vi "FGV Interference.vi"(0 "TestKonfig":T5={"TestKonfig H2O"={"Modus"=0, "Komponente:"=0, "Eingangs Konzentration:"=120.0, "Einheit"=enum."ppm", "Anzahl Stufen"=0.0, "Zeitdauer Stufen"=0.0, "Max Fehler"=0.0, "zusätzliche Zeitdauer Erster Punkt"=30.0, "Punkte umkehren"=FALSE, "Stufen Tabelle"=[], "HovaCAL Flow Input Cluster"={"HovaCAL Flow Input Cluster"=0.0}, "HovaCAL Temperature"=[]}, "TestKonfig Interferent"={"MFC1"=enum."MFC 1", "Eingangs Konzentration MFC1"=120.0, "Einheit MFC1 Eingang"=enum."ppm", "Ausgangs Konzentration MFC1"=120.0, "Einheit MFC1 Ausgang"=enum."ppm", "MFC2"=0, "Referenz-Interferent:"=0, "Gasflaschen Nr MFC2"="", "Eingangs Konzentration MFC2"=120.0, "Einheit MFC2 Eingang"=enum."ppm", "Accuracy MFC2"="", "Ausgangs Konzentration MFC2"=120.0, "Einheit MFC2 Ausgang"=enum."ppm", "MFC3"=1, "Kontroll-Interferent:"=0, "Gasflaschen Nr MFC3"="", "Accuracy MFC3"="", "Eingangs Konzentration MFC3"=120.0, "Einheit MFC3 Eingang"=enum."ppm", "Ausgangs Konzentration MFC3"=120.0, "Einheit MFC3 Ausgang"=enum."ppm", "Gasflasche MFC2"=0, "Gasflasche MFC3"=0}} {"TestKonfig Interferent"."Gasflasche MFC3" items=["----"=10000, "IAG NH3 3000"=0, "IAG NH3 200"=1, "IAG NH3 2000"=2, "IAG MG"=3, "IAG O2"=4]; "TestKonfig Interferent"."Gasflasche MFC2" items=["----"=10000, "IAG NH3 3000"=0, "IAG NH3 200"=1, "IAG NH3 2000"=2, "IAG MG"=3, "IAG O2"=4]; "TestKonfig Interferent"."Eingangs Konzentration MFC1" min=0.0; "TestKonfig Interferent"."Ausgangs Konzentration MFC1" min=0.0; "TestKonfig Interferent"."MFC2" items=["MFC 2", "MFC 3", "MFC 4", "MFC 5"]; "TestKonfig Interferent"."MFC3" items=["MFC 2", "MFC 3", "MFC 4", "MFC 5"]; "TestKonfig Interferent"."Ausgangs Konzentration MFC3" min=0.0; "TestKonfig Interferent"."Eingangs Konzentration MFC3" min=0.0; "TestKonfig Interferent"."Ausgangs Konzentration MFC2" min=0.0; "TestKonfig Interferent"."Eingangs Konzentration MFC2" min=0.0; "TestKonfig H2O"."HovaCAL Temperature" format="%.2f"; "TestKonfig H2O"."HovaCAL Flow Input Cluster"."HovaCAL Flow Input Cluster" format="%.2f"; "TestKonfig H2O"."Eingangs Konzentration:" min=0.0; "TestKonfig H2O"."zusätzliche Zeitdauer Erster Punkt" min=30 step=1 format="%#_5g"; "TestKonfig H2O"."Zeitdauer Stufen" format="%#_5g"; "TestKonfig H2O"."Max Fehler" format="%#_5g"; "TestKonfig H2O"."Anzahl Stufen" format="%#_5g"; "TestKonfig H2O"."Modus" items=["Messen", "CG zu Entnahmestelle"]}, 1 "TestSetting":T1={"Bearbeiter:"="", "Pfad:"=path "D:/IAG_Data/Log", "Textname:"="", "Analysator"=""}, 2 "Ergebnis":T4 caption="Ergebnis Cluster", 5 "Ergebnis":sgl[](array[numeric]), 7 "Einheiten":string[](array[string]), 9 "Tabelle":T3[][](array[typedef]), 11 "error in (no error)":errorcluster caption="Fehler (Eingang, kein Fehler)", 12 "Aktion FGV Interference":T15) -> (3 "TestSetting":T1={"Bearbeiter:"="", "Pfad:"=path "D:/IAG_Data/Log", "Textname:"="", "Analysator"=""}, 4 "TestKonfig":T5={"TestKonfig H2O"={"Modus"=0, "Komponente:"=0, "Eingangs Konzentration:"=120.0, "Einheit"=enum."ppm", "Anzahl Stufen"=0.0, "Zeitdauer Stufen"=0.0, "Max Fehler"=0.0, "zusätzliche Zeitdauer Erster Punkt"=30.0, "Punkte umkehren"=FALSE, "Stufen Tabelle"=[], "HovaCAL Flow Input Cluster"={"HovaCAL Flow Input Cluster"=0.0}, "HovaCAL Temperature"=[]}, "TestKonfig Interferent"={"MFC1"=enum."MFC 1", "Eingangs Konzentration MFC1"=120.0, "Einheit MFC1 Eingang"=enum."ppm", "Ausgangs Konzentration MFC1"=120.0, "Einheit MFC1 Ausgang"=enum."ppm", "MFC2"=0, "Referenz-Interferent:"=0, "Gasflaschen Nr MFC2"="", "Eingangs Konzentration MFC2"=120.0, "Einheit MFC2 Eingang"=enum."ppm", "Accuracy MFC2"="", "Ausgangs Konzentration MFC2"=120.0, "Einheit MFC2 Ausgang"=enum."ppm", "MFC3"=1, "Kontroll-Interferent:"=0, "Gasflaschen Nr MFC3"="", "Accuracy MFC3"="", "Eingangs Konzentration MFC3"=120.0, "Einheit MFC3 Eingang"=enum."ppm", "Ausgangs Konzentration MFC3"=120.0, "Einheit MFC3 Ausgang"=enum."ppm", "Gasflasche MFC2"=0, "Gasflasche MFC3"=0}} {"TestKonfig Interferent"."Gasflasche MFC3" items=["----"=10000, "IAG NH3 3000"=0, "IAG NH3 200"=1, "IAG NH3 2000"=2, "IAG MG"=3, "IAG O2"=4]; "TestKonfig Interferent"."Gasflasche MFC2" items=["----"=10000, "IAG NH3 3000"=0, "IAG NH3 200"=1, "IAG NH3 2000"=2, "IAG MG"=3, "IAG O2"=4]; "TestKonfig Interferent"."Eingangs Konzentration MFC1" min=0.0; "TestKonfig Interferent"."Ausgangs Konzentration MFC1" min=0.0; "TestKonfig Interferent"."MFC2" items=["MFC 2", "MFC 3", "MFC 4", "MFC 5"]; "TestKonfig Interferent"."MFC3" items=["MFC 2", "MFC 3", "MFC 4", "MFC 5"]; "TestKonfig Interferent"."Ausgangs Konzentration MFC3" min=0.0; "TestKonfig Interferent"."Eingangs Konzentration MFC3" min=0.0; "TestKonfig Interferent"."Ausgangs Konzentration MFC2" min=0.0; "TestKonfig Interferent"."Eingangs Konzentration MFC2" min=0.0; "TestKonfig H2O"."HovaCAL Temperature" format="%.2f"; "TestKonfig H2O"."HovaCAL Flow Input Cluster"."HovaCAL Flow Input Cluster" format="%.2f"; "TestKonfig H2O"."Eingangs Konzentration:" min=0.0; "TestKonfig H2O"."zusätzliche Zeitdauer Erster Punkt" min=30 step=1 format="%#_5g"; "TestKonfig H2O"."Zeitdauer Stufen" format="%#_5g"; "TestKonfig H2O"."Max Fehler" format="%#_5g"; "TestKonfig H2O"."Anzahl Stufen" format="%#_5g"; "TestKonfig H2O"."Modus" items=["Messen", "CG zu Entnahmestelle"]}, 6 "Ergebnis":T4, 8 "Einheiten":string[](array[string]), 10 "Tabelle":T3[][](array[typedef]), 15 "error out":errorcluster caption="Fehler (Ausgang)")   [LabVIEW 2020, in "EPA 1065.lvlib" / "HovaCAL Interference verificaton.lvlib"]
uses:
  HovaCAL Interference verificaton.lvlib
  Aktion FGV Interference.ctl
  TestKonfig.ctl
  TestKonfig H2O.ctl
  Modus.ctl
  Linearisierung V2/SpanEinstellungen/Einheit.ctl
  Linearisierung V2/Gasteiler/Stufen Tabelle.ctl
  Linearisierung V2/Gasteiler/HovaCAL_Interface/Controls/Flow Einstellung.ctl
  Linearisierung V2/Gasteiler/HovaCAL_Interface/Controls/Temp Sollwerte Anzeige.ctl
  TestKonfig Interferents.ctl
  MFCAuswahl.ctl
  Seiten/System Einstellungen V2/Gasflasche Auswahl.ctl
  Ergebnis.ctl
  Visualisierungs Elemente/String - Ausgabefeld.ctl
  TestSetting.ctl
  Seiten/System Einstellungen V2/Analysatoren.ctl
  Allgemein/allgemeine Sub-VIs.lvlib
  Seiten/System Einstellungen V2/System Einstellungen V2.lvlib
  Linearisierung V2/SpanEinstellungen/SpanEinstellungen.lvlib
  Linearisierung V2/Gasteiler/Gasteiler.lvlib
  Linearisierung V2/Gasteiler/HovaCAL_Interface/Controls/Controls.lvlib
panel:
  # "sec"
  # "%"
  # "sec"
  # "sec"
  # "%"
  # "sec"
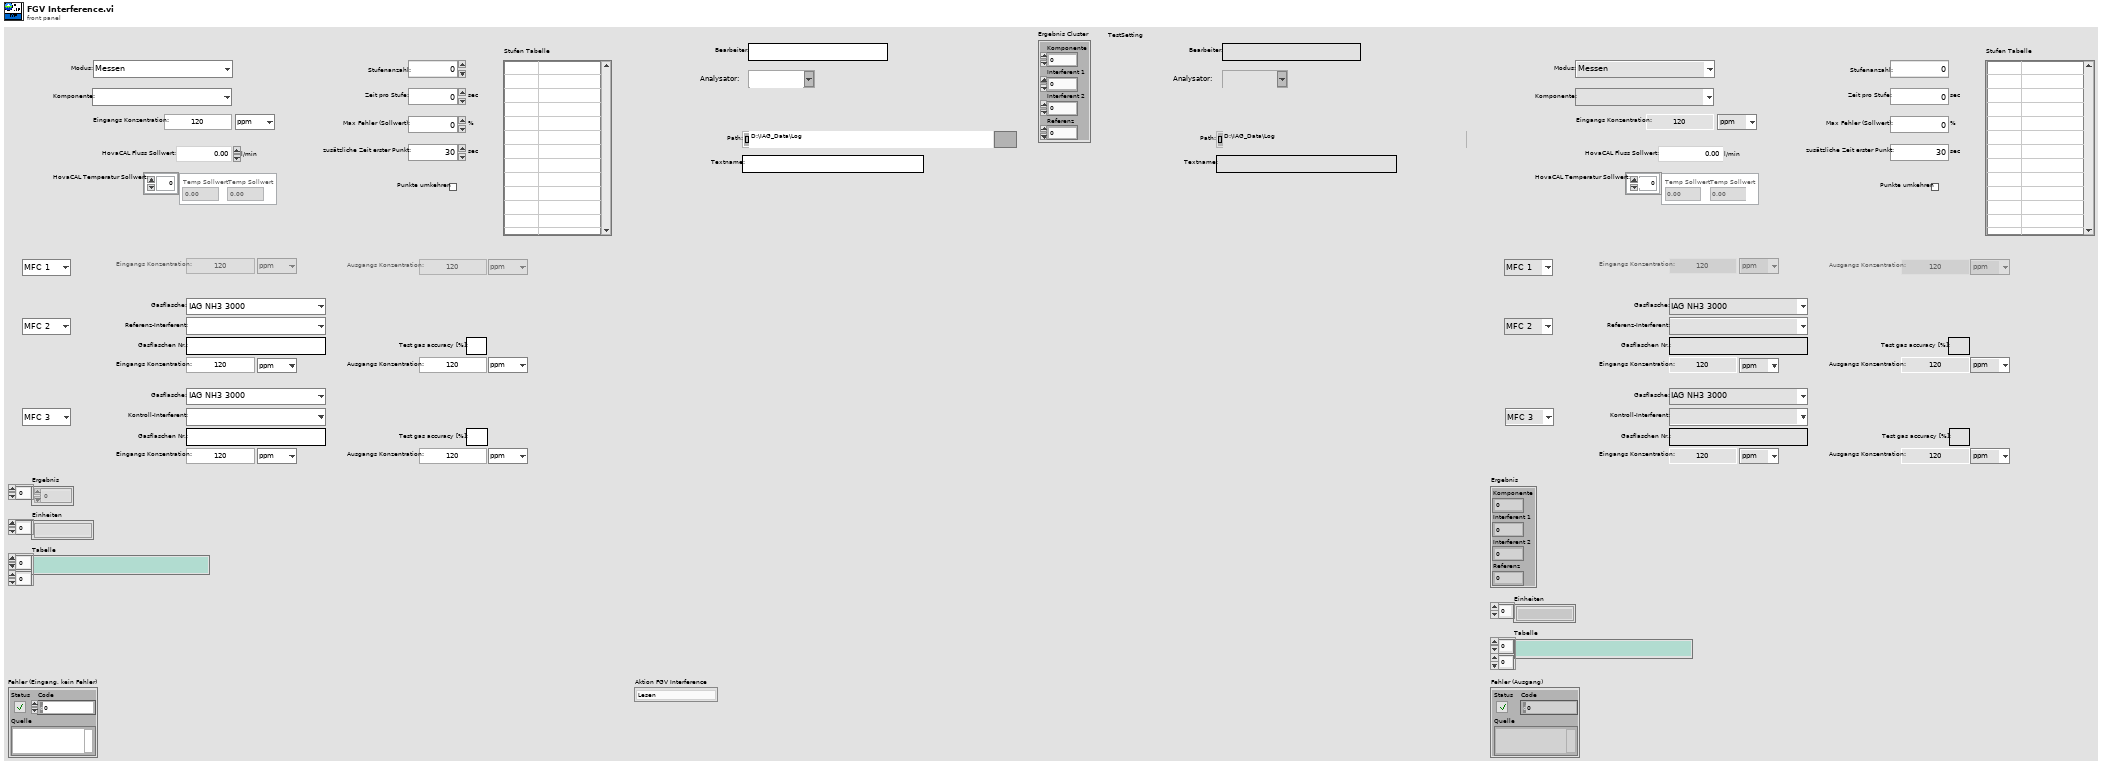
[diagram p1: front panel]
types:
  T1 = typedef "EPA 1065.lvlib/HovaCAL Interference verificaton.lvlib/TestSetting.ctl" = cluster{"Bearbeiter:":string, "Pfad:":path, "Textname:":string, "Analysator":T2}
  T2 = typedef "System Einstellungen V2.lvlib/Analysatoren.ctl" = string
  T3 = typedef "String - Ausgabefeld.ctl" = string
  T4 = typedef "EPA 1065.lvlib/HovaCAL Interference verificaton.lvlib/Ergebnis.ctl" = cluster{"Komponente":sgl, "Interferent 1":sgl, "Interferent 2":sgl, "Referenz":sgl}
  T5 = typedef "EPA 1065.lvlib/HovaCAL Interference verificaton.lvlib/TestKonfig.ctl" = cluster{"TestKonfig H2O":T6, "TestKonfig Interferent":T12}
  T6 = typedef "EPA 1065.lvlib/HovaCAL Interference verificaton.lvlib/TestKonfig H2O.ctl" = cluster{"Modus":T7, "Komponente:":u16, "Eingangs Konzentration:":dbl, "Einheit":T8, "Anzahl Stufen":sgl, "Zeitdauer Stufen":sgl, "Max Fehler":sgl, "zusätzliche Zeitdauer Erster Punkt":sgl, "Punkte umkehren":bool, "Stufen Tabelle":T9, "HovaCAL Flow Input Cluster":T10, "HovaCAL Temperature":T11}
  T7 = typedef "EPA 1065.lvlib/HovaCAL Interference verificaton.lvlib/Modus.ctl" = u16
  T8 = typedef "Linearisierung v2.lvlib/SpanEinstellungen.lvlib/Einheit.ctl" = enum16{"ppm", "%"}
  T9 = typedef "Linearisierung v2.lvlib/Gasteiler.lvlib/Stufen Tabelle.ctl" = string[][]
  T10 = typedef "Linearisierung v2.lvlib/Gasteiler.lvlib/HovaCAL_Interface.lvlib/Controls.lvlib/Flow Einstellung.ctl" = cluster{"HovaCAL Flow Input Cluster":dbl}
  T11 = typedef "Linearisierung v2.lvlib/Gasteiler.lvlib/HovaCAL_Interface.lvlib/Controls.lvlib/Temp Sollwerte Anzeige.ctl" = dbl[]
  T12 = typedef "EPA 1065.lvlib/HovaCAL Interference verificaton.lvlib/TestKonfig Interferents.ctl" = cluster{"MFC1":enum16{"MFC 1"}, "Eingangs Konzentration MFC1":dbl, "Einheit MFC1 Eingang":T8, "Ausgangs Konzentration MFC1":dbl, "Einheit MFC1 Ausgang":T8, "MFC2":T13, "Referenz-Interferent:":u16, "Gasflaschen Nr MFC2":string, "Eingangs Konzentration MFC2":dbl, "Einheit MFC2 Eingang":T8, "Accuracy MFC2":string, "Ausgangs Konzentration MFC2":dbl, "Einheit MFC2 Ausgang":T8, "MFC3":T13, "Kontroll-Interferent:":u16, "Gasflaschen Nr MFC3":string, "Accuracy MFC3":string, "Eingangs Konzentration MFC3":dbl, "Einheit MFC3 Eingang":T8, "Ausgangs Konzentration MFC3":dbl, "Einheit MFC3 Ausgang":T8, "Gasflasche MFC2":T14, "Gasflasche MFC3":T14}
  T13 = typedef "EPA 1065.lvlib/HovaCAL Interference verificaton.lvlib/MFCAuswahl.ctl" = u16
  T14 = typedef "System Einstellungen V2.lvlib/Gasflasche Auswahl.ctl" = u16
  T15 = typedef "EPA 1065.lvlib/HovaCAL Interference verificaton.lvlib/Aktion FGV Interference.ctl" = enum16{"Lesen", "TestKonfig", "TestSetting", "Einheiten", "Ergebnis", "Laden", "Tabelle", "Speichern", "löschen"}
  T16 = enum16{"open", "replace", "create", "open or create", "replace or create", "replace or create with confirmation"}
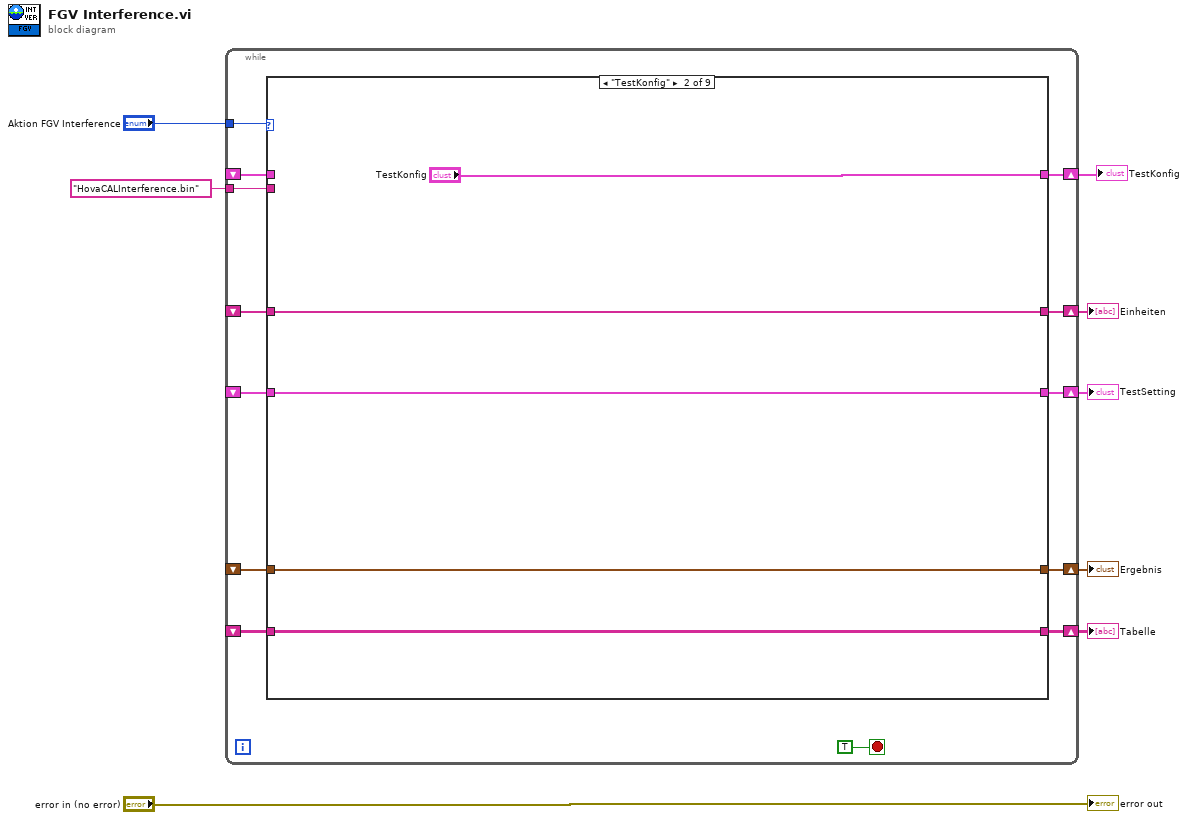
[diagram p0: block diagram]
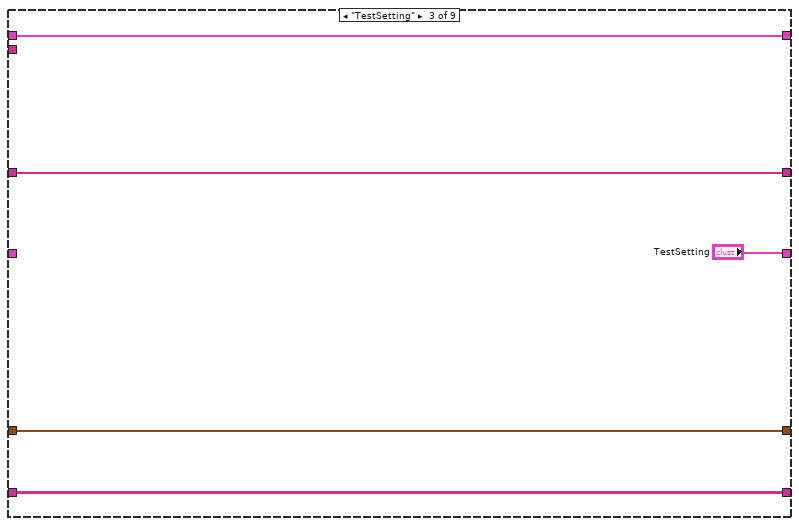
[diagram p3: hidden frame]
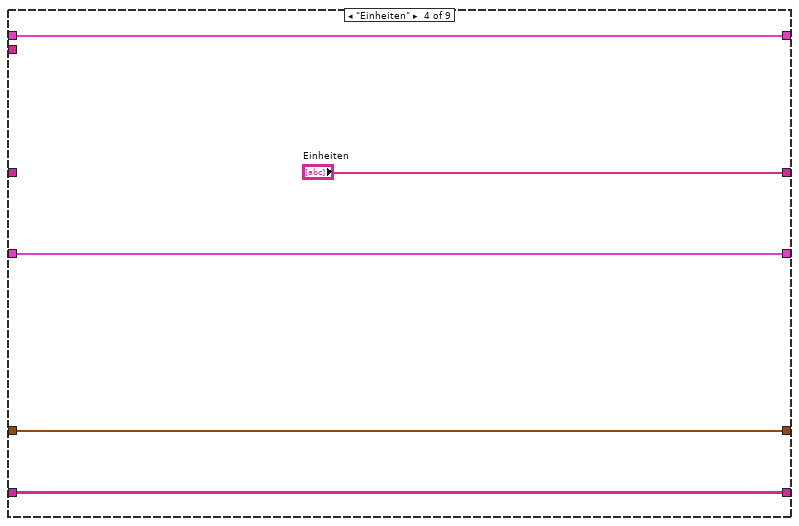
[diagram p4: hidden frame]
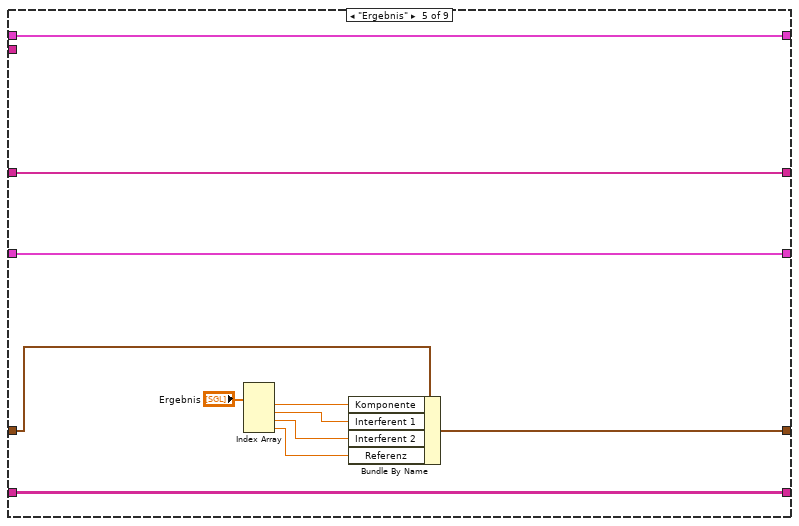
[diagram p5: hidden frame]
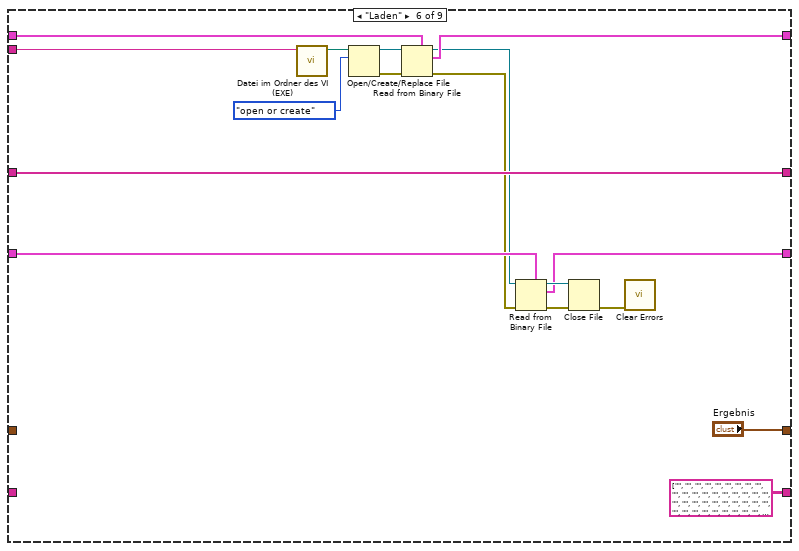
[diagram p6: hidden frame]
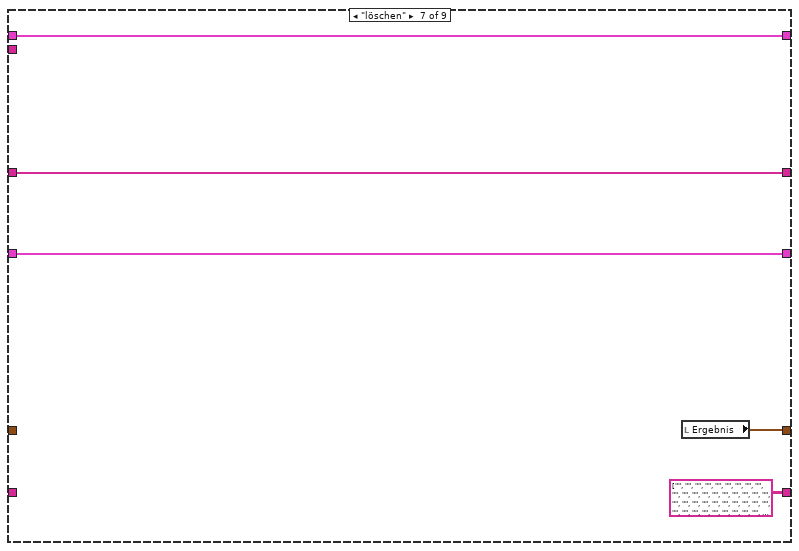
[diagram p7: hidden frame]
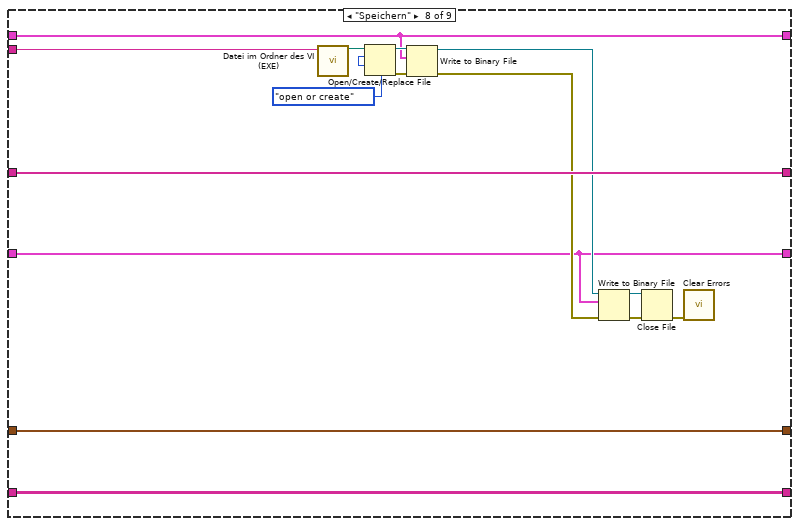
[diagram p8: hidden frame]
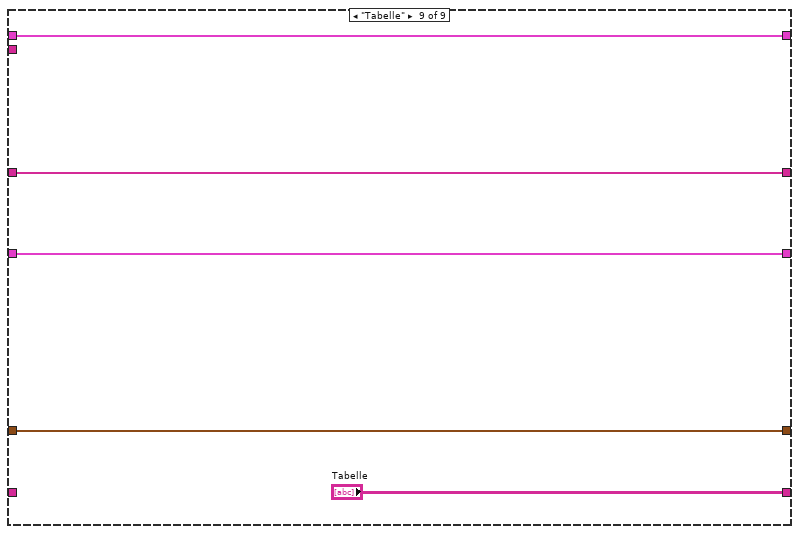
[diagram p9: hidden frame]
diagram:
  n1 = while {
    tunnel: "Aktion FGV Interference" -> [w20]
    shift-right: [w21] -> w6
    shift-left: _ -> [w19]
    shift-right: [w17] -> w5
    shift-left: _ -> [w16]
    shift-right: [w15] -> w4
    shift-left: _ -> [w14]
    shift-right: [w13] -> w3
    shift-left: _ -> [w12]
    shift-right: [w11] -> w2
    shift-left: _ -> [w10]
    tunnel: "HovaCALInterference.bin" ("Dateiname") -> [w9]
    stop <- TRUE stop-if-true
    n2 = case shown="\"TestKonfig\"" w20 {
      tunnel: [w26 "TestKonfig" w33 w41 w52 w61 w72 w82 w92] -> w21
      tunnel: w19 -> [w26 _ w33 w41 w52 w62 w72 w82 w92]
      tunnel: [w25 w30 w36 w40 w47 "Ergebnis" w71 w89 w94] -> w17
      tunnel: w16 -> [w25 w30 w36 w40 w50 _ _ w89 w94]
      tunnel: [w24 w29 w35 "Einheiten" w49 w68 w74 w88 w93] -> w15
      tunnel: w14 -> [w24 w29 w35 _ w49 w68 w74 w88 w93]
      tunnel: [w23 w28 w34 w38 w48 T3[][] [["", "", "", "", "", "", "", "", "", "", ""], ["", "", "", "", "", "", "", "", "", "", ""], ["", "", "", "", "", "", "", "", "", "", ""], ["", "", "", "", "", "", "", "", "", "", ""], ["", "", "", "", "", "", "", "", "", "", ""], ["", "", "", "", "", "", "", "", "", "", ""], ["", "", "", "", "", "", "", "", "", "", ""], ["", "", "", "", "", "", "", "", "", "", ""], ["", "", "", "", "", "", "", "", "", "", ""], ["", "", "", "", "", "", "", "", "", "", ""], ["", "", "", "", "", "", "", "", "", "", ""]] ("Tabelle") T3[][] [["", "", "", "", "", "", "", "", "", "", ""], ["", "", "", "", "", "", "", "", "", "", ""], ["", "", "", "", "", "", "", "", "", "", ""], ["", "", "", "", "", "", "", "", "", "", ""], ["", "", "", "", "", "", "", "", "", "", ""], ["", "", "", "", "", "", "", "", "", "", ""], ["", "", "", "", "", "", "", "", "", "", ""], ["", "", "", "", "", "", "", "", "", "", ""], ["", "", "", "", "", "", "", "", "", "", ""], ["", "", "", "", "", "", "", "", "", "", ""], ["", "", "", "", "", "", "", "", "", "", ""]] ("Tabelle") w87 "Tabelle"] -> w13
      tunnel: w12 -> [w23 w28 w34 w38 w48 _ _ w87 _]
      tunnel: [w22 w27 "TestSetting" w37 w46 w56 w70 w76 w91] -> w11
      tunnel: w10 -> [w22 w27 _ w37 w46 w57 w70 w76 w91]
      tunnel: w9 -> [_ _ _ _ _ w53 _ w75 _]
      frame "Lesen", Default {
      }
      frame "TestKonfig" {
      }
      frame "TestSetting" {
      }
      frame "Einheiten" {
      }
      frame "Ergebnis" {
        n3 = Index Array(array="Ergebnis") -> (element #1=w45:sgl, element #2=w44:sgl, element #3=w43:sgl, element #4=w42:sgl)  [unwired: 4 in]
        n4 = Bundle By Name(cluster=w50, "Komponente"=w45, "Interferent 1"=w44, "Interferent 2"=w43, "Referenz"=w42) -> (w47:T4)
      }
      frame "Laden" {
        n5 = call "Datei im Ordner des VI (EXE).vi"("Dateiname"=w53) -> ("Dateipfad im Ordner des Haupt-VIs"=w66:path)  [unwired: 8 in, 2 out]
        n6 = Open/Create/Replace File(file path (use dialog)=w66, operation (0:open)=T16."open or create" ("Operation (0:open)")) -> (refnum out=w64:refnum<file>, error out=w65:errorcluster)  [unwired: 4 in, 1 out]
        n7 = Read from Binary File(5:w62, 8:w65, 11:w64) -> (0:w54:errorcluster, 2:w61:T5, 3:w55:refnum<file>)  [unwired: 3 in, 1 out]
        n8 = Read from Binary File(5:w57, 8:w54, 11:w55) -> (0:w58:errorcluster, 2:w56:T1, 3:w60:refnum<file>)  [unwired: 3 in, 1 out]
        n9 = Close File(refnum=w60, error in=w58) -> (error out=w59:errorcluster)  [unwired: 1 out]
        n10 = call <vilib>:"Clear Errors.vi"("error in (no error)"=w59) -> ()  [unwired: 5 in, 2 out]
      }
      frame "löschen" {
        n11 = local read "Ergebnis"() -> (w71:T4)
      }
      frame "Speichern" {
        n12 = call "Datei im Ordner des VI (EXE).vi"("Dateiname"=w75) -> ("Dateipfad im Ordner des Haupt-VIs"=w85:path)  [unwired: 8 in, 2 out]
        n13 = Open/Create/Replace File(file path (use dialog)=w85, operation (0:open)=T16."open or create" ("Operation (0:open)")) -> (refnum out=w86:refnum<file>, error out=w84:errorcluster)  [unwired: 4 in, 1 out]
        n14 = Write to Binary File(file (use dialog)=w86, data=w82, error in=w84) -> (refnum out=w78:refnum<file>, error out=w77:errorcluster)  [unwired: 3 in, 1 out]
        n15 = Write to Binary File(file (use dialog)=w78, data=w76, error in=w77) -> (refnum out=w80:refnum<file>, error out=w81:errorcluster)  [unwired: 3 in, 1 out]
        n16 = Close File(refnum=w80, error in=w81) -> (error out=w79:errorcluster)  [unwired: 1 out]
        n17 = call <vilib>:"Clear Errors.vi"("error in (no error)"=w79) -> ()  [unwired: 5 in, 2 out]
      }
      frame "Tabelle" {
      }
    }
  }
  "TestKonfig" <- w6
  "Ergebnis" <- w5
  "Einheiten" <- w4
  "Tabelle" <- w3
  "TestSetting" <- w2
  "error out" <- "error in (no error)"
